vi "Teleop.vi"(10 "Match Info":T1={"Autonomous Elapsed Seconds"=0.0, "TeleOp Elapsed Seconds"=0.0, "Disabled Elapsed Seconds"=0.0, "Visited Autonomous"=FALSE, "Visited TeleOp"=FALSE, "Visited Disabled"=FALSE, "Autonomous Settings"={"Autonomous Style"=enum."Independent", "VI Refnum"=refnum}}, 11 "Call Context":T2) -> ()   [LabVIEW 2012]
doc: "This VI is called for each TeleOp packet received from the DS where the robot is not disabled. It is often used to read from the joysticks and update I/O or to update setpoints for timed control loops. It should complete and return within 20 milliseconds or it may miss DS packets."
uses:
  <vilib>/Rock Robotics/WPI/DriverStation/WPI_DriverStationDerivedRobotMode.ctl
  <vilib>/Rock Robotics/WPI/DriverStation/WPI_DriverStationMatch Info.ctl
  <vilib>/Rock Robotics/WPI/Relay/WPI_RelayValue.ctl
  Robot Global Data.vi
  <vilib>/Rock Robotics/WPI/Joystick/WPI_JoystickGetSetRefNum.vi
panel:
  in  "Ext Const":dbl=0.5
  in  "Dep Const":dbl=1.0
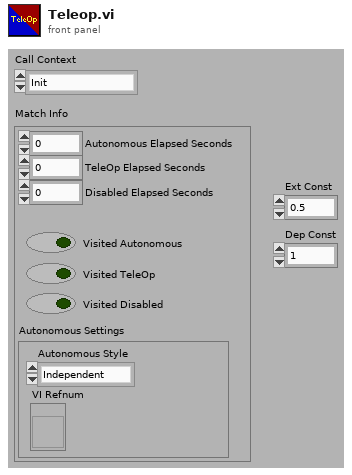
[diagram p1: front panel]
types:
  T1 = typedef "WPI_DriverStationMatch Info.ctl" = cluster{"Autonomous Elapsed Seconds":dbl, "TeleOp Elapsed Seconds":dbl, "Disabled Elapsed Seconds":dbl, "Visited Autonomous":bool, "Visited TeleOp":bool, "Visited Disabled":bool, "Autonomous Settings":cluster{"Autonomous Style":enum16{"Iterative", "Independent"}, "VI Refnum":refnum<vi>}}
  T2 = typedef "WPI_DriverStationDerivedRobotMode.ctl" = enum16{"Init", "Execute", "Stop"}
  T3 = typedef "WPI_RelayValue.ctl" = enum16{"Off", "On", "Forward", "Reverse"}
  T4 = cluster{"Driver Station Digital Input (1-8)[0]":bool, "Driver Station Digital Input (1-8)[1]":bool, "Driver Station Digital Input (1-8)[2]":bool, "Driver Station Digital Input (1-8)[3]":bool, "Driver Station Digital Input (1-8)[4]":bool, "Driver Station Digital Input (1-8)[5]":bool, "Driver Station Digital Input (1-8)[6]":bool, "Driver Station Digital Input (1-8)[7]":bool, "Driver Station Digital Input (1-8)[8]":bool}
  T5 = cluster{"Right Servo High":dbl, "Right Servo Mid":dbl, "Right Servo Low":dbl, "Left Servo High":dbl, "Left Servo Mid":dbl, "Left Servo Low":dbl}
  T6 = typedef "WPI_DigitalInputDevRef.ctl" = cluster{"DevStatus":errorcluster, "DIO Channel":T7, "Digital Module":T8}
  T7 = typedef "FPGA_DIOChannel.ctl" = enum8{"DIO 1", "DIO 2", "DIO 3", "DIO 4", "DIO 5", "DIO 6", "DIO 7", "DIO 8", "DIO 9", "DIO 10", "DIO 11", "DIO 12", "DIO 13", "DIO 14", "Invalid"}
  T8 = typedef "FPGA_TypedefDigitalModule.ctl" = enum16{"Digital Module 1", "Digital Module 2"}
  T9 = typedef "WPI_JoystickDevRef.ctl" = cluster{"Device":T10}
  T10 = typedef "WPI_JoystickDeviceEnum.ctl" = enum16{"USB 1", "USB 2", "USB 3", "USB 4", "Kinect 1", "Kinect 2"}
  T11 = cluster{"axis 1 (x)":dbl, "axis 2 (y)":dbl, "axis 3 (throttle)":dbl, "axis 4":dbl, "axis 5":dbl, "axis 6":dbl}
  T12 = typedef "WPI_RelayDevRef.ctl" = cluster{"DevStatus":errorcluster, "Relay Channel":T13, "Digital Module":T8, "Relay Direction":T14}
  T13 = typedef "FPGA_DIORelayChannel.ctl" = enum8{"Relay 1", "Relay 2", "Relay 3", "Relay 4", "Relay 5", "Relay 6", "Relay 7", "Relay 8", "Invalid"}
  T14 = typedef "WPI_RelayDirection.ctl" = enum16{"Both directions", "Forward only", "Reverse only"}
  T15 = typedef "WPI_ServoDeviceRef.ctl" = cluster{"DeviceStatus":errorcluster, "Digital Module":T8, "PWM Channel":T16, "DeadBand":T17}
  T16 = typedef "FPGA_DIOPWMChannel.ctl" = enum8{"PWM 1", "PWM 2", "PWM 3", "PWM 4", "PWM 5", "PWM 6", "PWM 7", "PWM 8", "PWM 9", "PWM 10", "Invalid"}
  T17 = typedef "WPI_PWMDeadband.ctl" = cluster{"Name":string, "maxPositivePwm":i32, "minPositivePwm":i32, "centerPwm":i32, "maxNegativePwm":i32, "minNegativePwm":i32, "angularRange":u16}
  T18 = typedef "WPI_MotorControlDeviceRef.ctl" = cluster{"DeviceStatus":errorcluster, "Type":enum16{"PWM", "CAN"}, "PWM":cluster{"Digital Module":T8, "PWM Channel":T16, "DeadBand":T17}, "CAN":cluster{"Device Number":u8, "Control Mode":T19, "Semaphore":T20, "Max Vout":dbl}, "Invert":bool, "TransformRef":T21, "InvTransformRef":T21}
  T19 = typedef "WPI_CANJaguar_ControlMode.ctl" = enum8{"Percent VBus", "Current", "Speed", "Position", "Voltage"}
  T20 = typedef "Semaphore RefNum" = refnum<k1>
  T21 = typedef "WPI_PWMTransform_ConPane.ctl" = refnum<vi>
  T22 = typedef "WPI_JoystickButtonState.ctl" = cluster{"Button 1":bool, "Button 2":bool, "Button 3":bool, "Button 4":bool, "Button 5":bool, "Button 6":bool, "Button 7":bool, "Button 8":bool, "Button 9":bool, "Button 10":bool, "Button 11":bool, "Button 12":bool}
  T23 = cluster{"FlipperLeftUp":dbl, "FlipperLeftDown":dbl, "FlipperRightUp":dbl, "FlipperRightDown":dbl, "KickerLeftBack":dbl, "KickerLeftForward":dbl, "KickerRightBack":dbl, "KickerRightForward":dbl}
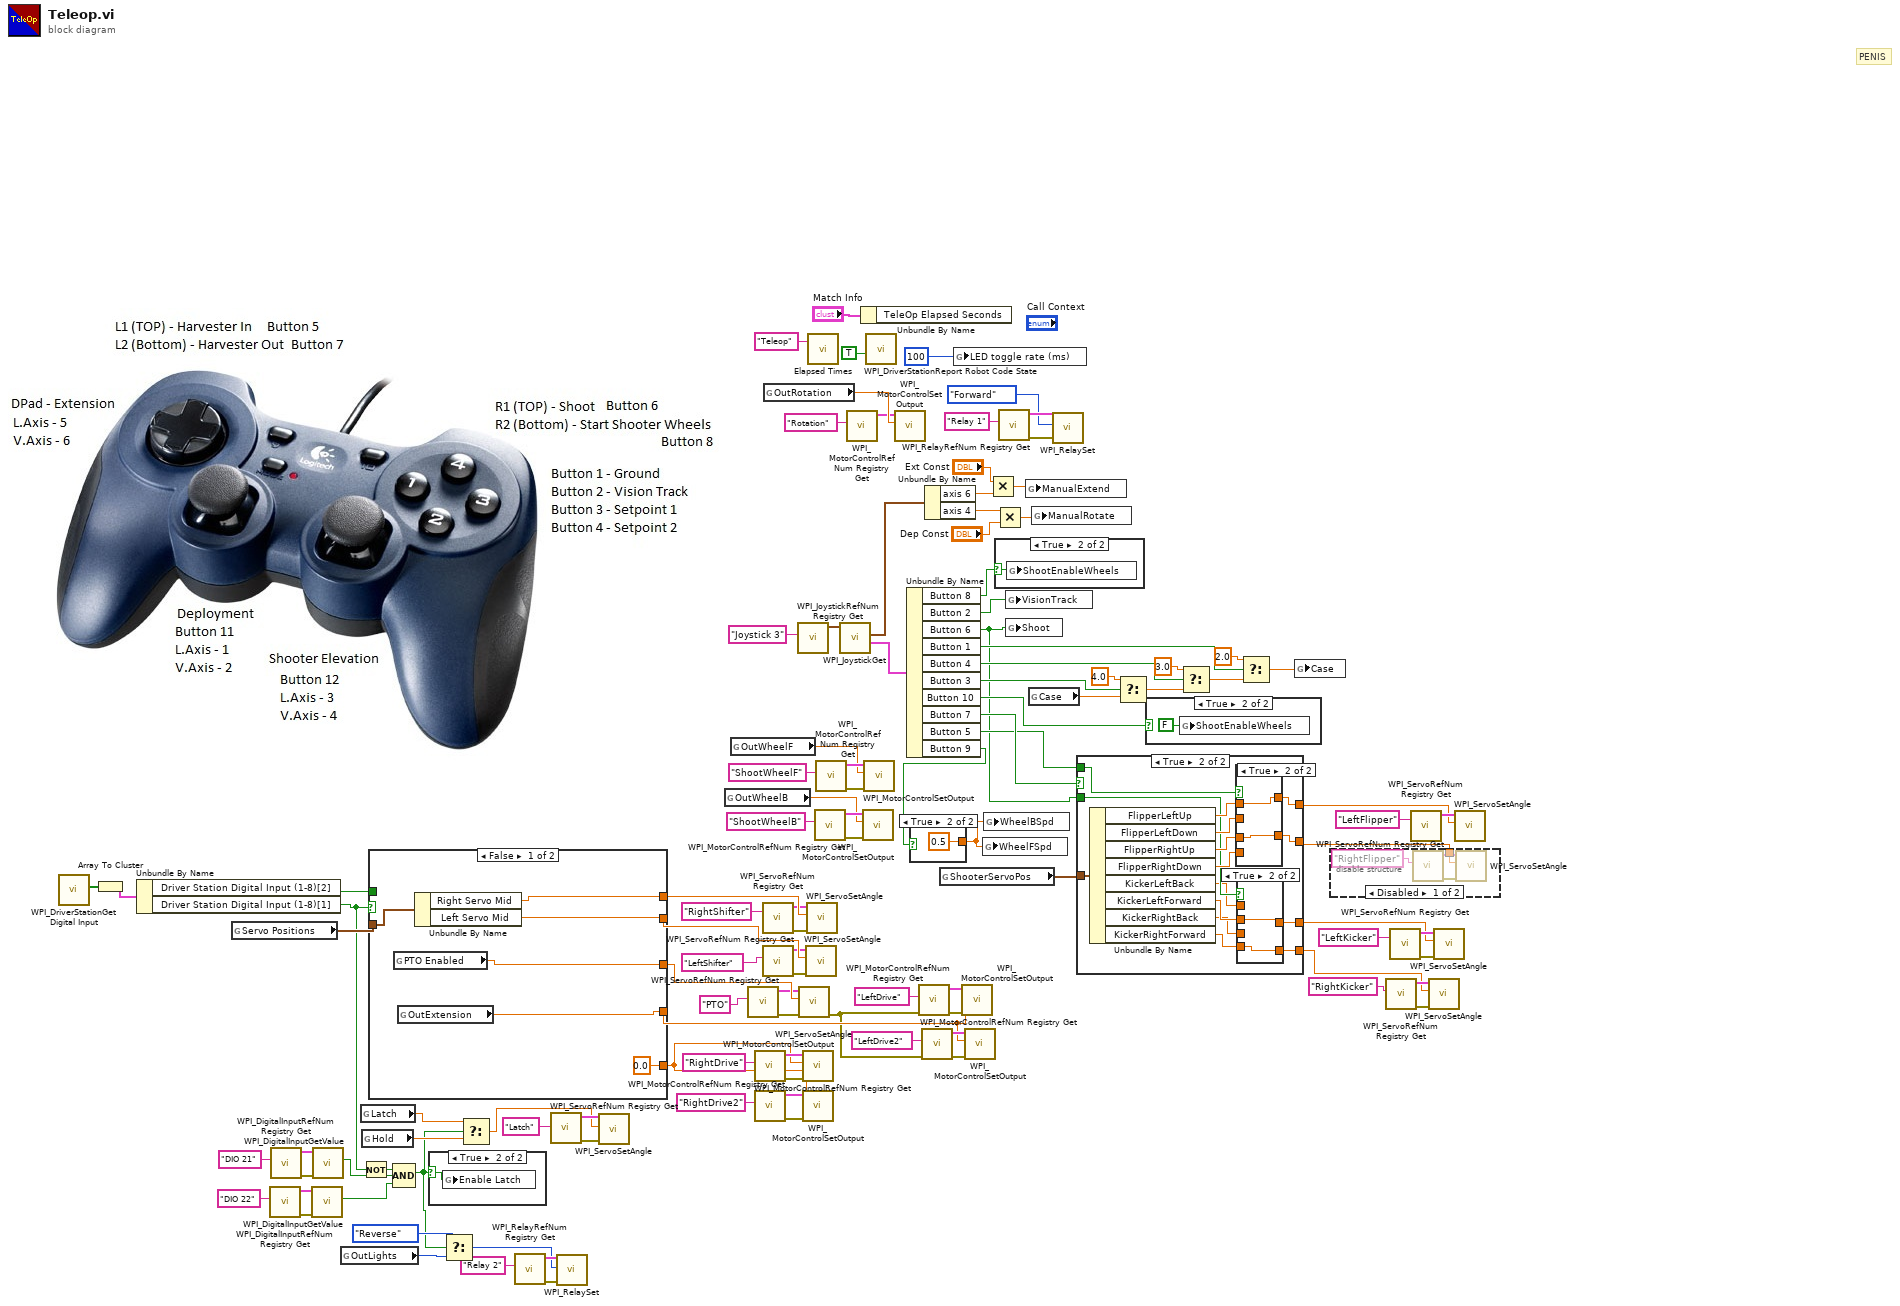
[diagram p0: block diagram]
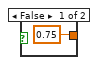
[diagram p2: hidden frame]
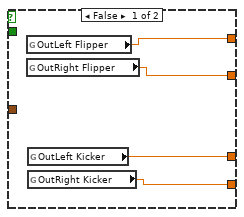
[diagram p4: hidden frame]
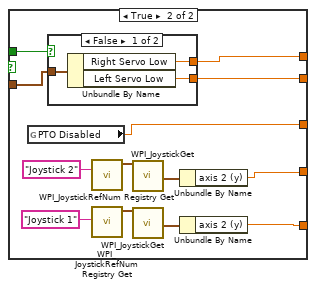
[diagram p8: hidden frame]
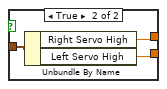
[diagram p9: hidden frame]
diagram:
  # "PENIS"
  n1 = call <vilib>:"WPI_DriverStationGet Digital Input.vi"() -> ("Driver Station Digital Input (1-8)"=w82:bool[])  [unwired: 11 in]
  n2 = Array To Cluster(array=w82) -> (cluster=w81:T4)
  n3 = Unbundle By Name(w81) -> ("Driver Station Digital Input (1-8)[2]"=w80:bool, "Driver Station Digital Input (1-8)[1]"=w41:bool)
  n4 = global read "Robot Global Data.vi" "Servo Positions"() -> (w79:T5)
  n5 = call <vilib>:"WPI_DigitalInputRefNum Registry Get.vi"("refnum name"="DIO 22") -> ("error out"=w5:errorcluster, "DigitalInputDevRef"=w6:T6)  [unwired: 9 in]
  n6 = call <vilib>:"WPI_DigitalInputRefNum Registry Get.vi"("refnum name"="DIO 21") -> ("error out"=w10:errorcluster, "DigitalInputDevRef"=w9:T6)  [unwired: 9 in]
  n7 = call <vilib>:"WPI_DigitalInputGetValue.vi"("error in (no error)"=w5, "DigitalInputDevRef"=w6) -> ("Value"=w2:bool)  [unwired: 7 in, 2 out]
  n8 = call <vilib>:"WPI_DigitalInputGetValue.vi"("error in (no error)"=w10, "DigitalInputDevRef"=w9) -> ("Value"=w3:bool)  [unwired: 7 in, 2 out]
  n9 = global read "Robot Global Data.vi" "OutLights"() -> (w47:T3)
  n10 = global read "Robot Global Data.vi" "Latch"() -> (w14:dbl)
  n11 = Not(x=w41) -> (.not. x?=w4:bool)
  n12 = global read "Robot Global Data.vi" "Hold"() -> (w13:dbl)
  n13 = case shown="False" w41 {
    tunnel: w80 -> [_ w133]
    tunnel: w79 -> [w120 w132]
    tunnel: [w119 w131] -> w78
    tunnel: [w118 w130] -> w77
    tunnel: [w117 w129] -> w70
    tunnel: [w115 w122] -> w69
    tunnel: [0.0 w121] -> w68
    frame False {
      n14 = global read "Robot Global Data.vi" "PTO Enabled"() -> (w117:dbl)
      n15 = global read "Robot Global Data.vi" "OutExtension"() -> (w115:dbl)
      n16 = Unbundle By Name(w120) -> ("Right Servo Mid"=w119:dbl, "Left Servo Mid"=w118:dbl)
    }
    frame True {
      n17 = global read "Robot Global Data.vi" "PTO Disabled"() -> (w129:dbl)
      n18 = case shown="False" w133 {
        tunnel: w132 -> [w136 w139]
        tunnel: [w135 w138] -> w131
        tunnel: [w134 w137] -> w130
        frame False {
          n19 = Unbundle By Name(w136) -> ("Right Servo Low"=w135:dbl, "Left Servo Low"=w134:dbl)
        }
        frame True {
          n20 = Unbundle By Name(w139) -> ("Right Servo High"=w138:dbl, "Left Servo High"=w137:dbl)
        }
      }
      n21 = call <vilib>:"WPI_JoystickRefNum Registry Get.vi"("refnum name"="Joystick 2") -> ("JoystickDevRef"=w123:T9)  [unwired: 1 in, 9 out]
      n22 = call <vilib>:"WPI_JoystickRefNum Registry Get.vi"("refnum name"="Joystick 1") -> ("JoystickDevRef"=w127:T9)  [unwired: 1 in, 9 out]
      n23 = call <vilib>:"WPI_JoystickGet.vi"("JoystickDevRef"=w123) -> ("Axes"=w125:T11)  [unwired: 1 in, 5 out]
      n24 = call <vilib>:"WPI_JoystickGet.vi"("JoystickDevRef"=w127) -> ("Axes"=w128:T11)  [unwired: 1 in, 5 out]
      n25 = Unbundle By Name(w125) -> ("axis 2 (y)"=w122:dbl)
      n26 = Unbundle By Name(w128) -> ("axis 2 (y)"=w121:dbl)
    }
  }
  n27 = Compound Arithmetic op=AND(w4, w3, w2) -> (w1:bool)
  n28 = case shown="True" w1 {
    selector: w1 -> [_ w140]
    frame False {
    }
    frame True {
      n29 = global write "Robot Global Data.vi" "Enable Latch"(w140) -> ()
    }
  }
  n30 = Select(t=WPI_RelayValue."Reverse" ("RelayValue"), s=w1, f=w47) -> (s? t:f=w45:T3)
  n31 = Select(t=w14, s=w1, f=w13) -> (s? t:f=w40:dbl)
  n32 = call <vilib>:"WPI_RelayRefNum Registry Get.vi"("refnum name"="Relay 2") -> ("error out"=w53:errorcluster, "RelayDevRef"=w51:T12)  [unwired: 9 in]
  n33 = call <vilib>:"WPI_ServoRefNum Registry Get.vi"("refnum name"="Latch") -> ("error out"=w44:errorcluster, "ServoDeviceRef"=w42:T15)  [unwired: 9 in]
  n34 = call <vilib>:"WPI_RelaySet.vi"("error in (no error)"=w53, "RelayValue"=w45, "RelayDevRef"=w51) -> ()  [unwired: 7 in, 2 out]
  n35 = call <vilib>:"WPI_ServoSetAngle.vi"("error in (no error)"=w44, "Angle"=w40, "ServoDeviceRef"=w42) -> ()  [unwired: 7 in, 2 out]
  n36 = global read "Robot Global Data.vi" "OutWheelB"() -> (w32:dbl)
  n37 = global read "Robot Global Data.vi" "OutWheelF"() -> (w33:dbl)
  n38 = call <vilib>:"WPI_ServoRefNum Registry Get.vi"("refnum name"="PTO") -> ("error out"=w63:errorcluster, "ServoDeviceRef"=w64:T15)  [unwired: 9 in]
  n39 = call <vilib>:"WPI_MotorControlRefNum Registry Get.vi"("refnum name"="RightDrive") -> ("error out"=w92:errorcluster, "MotorControlDevRef"=w94:T18)  [unwired: 9 in]
  n40 = call <vilib>:"WPI_MotorControlRefNum Registry Get.vi"("refnum name"="RightDrive2") -> ("error out"=w85:errorcluster, "MotorControlDevRef"=w83:T18)  [unwired: 9 in]
  n41 = call <vilib>:"WPI_ServoRefNum Registry Get.vi"("refnum name"="RightShifter") -> ("error out"=w73:errorcluster, "ServoDeviceRef"=w74:T15)  [unwired: 9 in]
  n42 = call <vilib>:"WPI_ServoRefNum Registry Get.vi"("refnum name"="LeftShifter") -> ("error out"=w75:errorcluster, "ServoDeviceRef"=w76:T15)  [unwired: 9 in]
  n43 = global read "Robot Global Data.vi" "OutRotation"() -> (w67:dbl)
  n44 = call <vilib>:"WPI_JoystickRefNum Registry Get.vi"("refnum name"="Joystick 3") -> ("JoystickDevRef"=w111:T9)  [unwired: 9 in, 1 out]
  n45 = call <vilib>:"WPI_ServoSetAngle.vi"("error in (no error)"=w63, "Angle"=w70, "ServoDeviceRef"=w64) -> ("error out"=w59:errorcluster)  [unwired: 7 in, 1 out]
  n46 = call <vilib>:"WPI_MotorControlSetOutput.vi"("error in (no error)"=w92, "Output"=w68, "MotorControlDevRef"=w94) -> ()  [unwired: 6 in, 3 out]
  n47 = call <vilib>:"WPI_MotorControlSetOutput.vi"("error in (no error)"=w85, "Output"=w68, "MotorControlDevRef"=w83) -> ()  [unwired: 6 in, 3 out]
  n48 = call <vilib>:"WPI_ServoSetAngle.vi"("error in (no error)"=w75, "Angle"=w77, "ServoDeviceRef"=w76) -> ()  [unwired: 7 in, 2 out]
  n49 = call <vilib>:"WPI_ServoSetAngle.vi"("error in (no error)"=w73, "Angle"=w78, "ServoDeviceRef"=w74) -> ()  [unwired: 7 in, 2 out]
  n50 = call "Elapsed Times.vi"("Call Name"="Teleop") -> ()  [unwired: 2 in, 1 out]
  n51 = call <vilib>:"WPI_MotorControlRefNum Registry Get.vi"("refnum name"="ShootWheelB") -> ("error out"=w35:errorcluster, "MotorControlDevRef"=w36:T18)  [unwired: 9 in]
  n52 = call <vilib>:"WPI_MotorControlRefNum Registry Get.vi"("refnum name"="ShootWheelF") -> ("error out"=w37:errorcluster, "MotorControlDevRef"=w34:T18)  [unwired: 9 in]
  n53 = call <vilib>:"WPI_JoystickGet.vi"("JoystickDevRef"=w111) -> ("Buttons"=w109:T22, "Axes"=w108:T11)  [unwired: 4 in, 1 out]
  n54 = call <vilib>:"WPI_MotorControlRefNum Registry Get.vi"("refnum name"="Rotation") -> ("MotorControlDevRef"=w65:T18)  [unwired: 9 in, 1 out]
  n55 = Unbundle By Name("Match Info") -> ()  [unwired: 1 out]
  n56 = call <vilib>:"WPI_MotorControlSetOutput.vi"("error in (no error)"=w35, "Output"=w32, "MotorControlDevRef"=w36) -> ()  [unwired: 6 in, 3 out]
  n57 = call <vilib>:"WPI_MotorControlSetOutput.vi"("error in (no error)"=w37, "Output"=w33, "MotorControlDevRef"=w34) -> ()  [unwired: 6 in, 3 out]
  n58 = call <vilib>:"WPI_DriverStationReport Robot Code State.vi"("TeleOp"=TRUE ("Autonomous")) -> ()  [unwired: 10 in, 1 out]
  n59 = call <vilib>:"WPI_MotorControlSetOutput.vi"("Output"=w67, "MotorControlDevRef"=w65) -> ()  [unwired: 7 in, 3 out]
  n60 = Unbundle By Name(w109) -> ("Button 8"=w96:bool, "Button 2"=w107:bool, "Button 6"=w16:bool, "Button 1"=w106:bool, "Button 4"=w104:bool, "Button 3"=w103:bool, "Button 10"=w31:bool, "Button 7"=w30:bool, "Button 5"=w29:bool, "Button 9"=w11:bool)
  n61 = case shown="True" w11 {
    tunnel: [0.75 0.5] -> w12
    frame False {
    }
    frame True {
    }
  }
  n62 = call <vilib>:"WPI_MotorControlRefNum Registry Get.vi"("error in (no error)"=w59, "refnum name"="LeftDrive") -> ("error out"=w87:errorcluster, "MotorControlDevRef"=w90:T18)  [unwired: 8 in]
  n63 = call <vilib>:"WPI_MotorControlRefNum Registry Get.vi"("error in (no error)"=w59, "refnum name"="LeftDrive2") -> ("error out"=w86:errorcluster, "MotorControlDevRef"=w88:T18)  [unwired: 8 in]
  n64 = Unbundle By Name(w108) -> ("axis 6"=w50:dbl, "axis 4"=w60:dbl)
  n65 = global read "Robot Global Data.vi" "ShooterServoPos"() -> (w17:T23)
  n66 = global write "Robot Global Data.vi" "LED toggle rate (ms)"(u32 100 ("LED ms toggle rate")) -> ()
  n67 = call <vilib>:"WPI_MotorControlSetOutput.vi"("error in (no error)"=w87, "Output"=w69, "MotorControlDevRef"=w90) -> ()  [unwired: 6 in, 3 out]
  n68 = call <vilib>:"WPI_MotorControlSetOutput.vi"("error in (no error)"=w86, "Output"=w69, "MotorControlDevRef"=w88) -> ()  [unwired: 6 in, 3 out]
  n69 = global write "Robot Global Data.vi" "WheelFSpd"(w12) -> ()
  n70 = global write "Robot Global Data.vi" "WheelBSpd"(w12) -> ()
  n71 = Multiply(x="Ext Const", y=w50) -> (x*y=w48:dbl)
  n72 = Multiply(x=w60, y="Dep Const") -> (x*y=w58:dbl)
  n73 = case shown="True" w96 {
    selector: w96 -> [_ w143]
    frame False {
    }
    frame True {
      n74 = global write "Robot Global Data.vi" "ShootEnableWheels"(w143) -> ()
    }
  }
  n75 = call <vilib>:"WPI_RelayRefNum Registry Get.vi"("refnum name"="Relay 1") -> ("error out"=w55:errorcluster, "RelayDevRef"=w57:T12)  [unwired: 9 in]
  n76 = global write "Robot Global Data.vi" "VisionTrack"(w107) -> ()
  n77 = global write "Robot Global Data.vi" "Shoot"(w16) -> ()
  n78 = global write "Robot Global Data.vi" "ManualExtend"(w48) -> ()
  n79 = global read "Robot Global Data.vi" "Case"() -> (w98:dbl)
  n80 = global write "Robot Global Data.vi" "ManualRotate"(w58) -> ()
  n81 = call <vilib>:"WPI_RelaySet.vi"("error in (no error)"=w55, "RelayValue"=WPI_RelayValue."Forward", "RelayDevRef"=w57) -> ()  [unwired: 7 in, 2 out]
  n82 = case shown="True" w30 {
    tunnel: w29 -> [_ w148]
    tunnel: [w147 w161] -> w20
    tunnel: [w146 w159] -> w19
    tunnel: [w145 w150] -> w18
    tunnel: [w144 w149] -> w15
    tunnel: w17 -> [_ w162]
    tunnel: w16 -> [_ w155]
    frame False {
      n83 = global read "Robot Global Data.vi" "OutLeft Flipper"() -> (w147:dbl)
      n84 = global read "Robot Global Data.vi" "OutRight Flipper"() -> (w146:dbl)
      n85 = global read "Robot Global Data.vi" "OutLeft Kicker"() -> (w145:dbl)
      n86 = global read "Robot Global Data.vi" "OutRight Kicker"() -> (w144:dbl)
    }
    frame True {
      n87 = Unbundle By Name(w162) -> ("FlipperLeftUp"=w160:dbl, "FlipperLeftDown"=w157:dbl, "FlipperRightUp"=w158:dbl, "FlipperRightDown"=w156:dbl, "KickerLeftBack"=w154:dbl, "KickerLeftForward"=w153:dbl, "KickerRightBack"=w152:dbl, "KickerRightForward"=w151:dbl)
      n88 = case shown="True" w148 {
        tunnel: [w168 w170] -> w161
        tunnel: w160 -> [_ w170]
        tunnel: [w167 w169] -> w159
        tunnel: w158 -> [_ w169]
        tunnel: w157 -> [w168 _]
        tunnel: w156 -> [w167 _]
        frame False {
        }
        frame True {
        }
      }
      n89 = case shown="True" w155 {
        tunnel: w154 -> [w164 _]
        tunnel: w153 -> [_ w165]
        tunnel: w152 -> [w163 _]
        tunnel: w151 -> [_ w166]
        tunnel: [w164 w165] -> w150
        tunnel: [w163 w166] -> w149
        frame False {
        }
        frame True {
        }
      }
    }
  }
  n90 = Select(t=4.0, s=w103, f=w98) -> (s? t:f=w102:dbl)
  n91 = case shown="True" w31 {
    frame False {
    }
    frame True {
      n92 = global write "Robot Global Data.vi" "ShootEnableWheels"(FALSE ("ShootStartWheels")) -> ()
    }
  }
  n93 = Select(t=3.0, s=w104, f=w102) -> (s? t:f=w100:dbl)
  n94 = Select(t=2.0, s=w106, f=w100) -> (s? t:f=w97:dbl)
  n95 = global write "Robot Global Data.vi" "Case"(w97) -> ()
  n96 = disable-structure shown="Disabled" {
    disable-tunnel: w19 -> [w172 _]
    frame Disabled {
      n97 = call <vilib>:"WPI_ServoRefNum Registry Get.vi"("refnum name"="RightFlipper") -> ("error out"=w175:errorcluster, "ServoDeviceRef"=w173:T15)  [unwired: 9 in]
      n98 = call <vilib>:"WPI_ServoSetAngle.vi"("error in (no error)"=w175, "Angle"=w172, "ServoDeviceRef"=w173) -> ()  [unwired: 7 in, 2 out]
    }
    frame Enabled {
    }
  }
  n99 = call <vilib>:"WPI_ServoRefNum Registry Get.vi"("refnum name"="RightKicker") -> ("error out"=w27:errorcluster, "ServoDeviceRef"=w25:T15)  [unwired: 9 in]
  n100 = call <vilib>:"WPI_ServoRefNum Registry Get.vi"("refnum name"="LeftKicker") -> ("error out"=w21:errorcluster, "ServoDeviceRef"=w22:T15)  [unwired: 9 in]
  n101 = call <vilib>:"WPI_ServoRefNum Registry Get.vi"("refnum name"="LeftFlipper") -> ("ServoDeviceRef"=w23:T15)  [unwired: 9 in, 1 out]
  n102 = call <vilib>:"WPI_ServoSetAngle.vi"("error in (no error)"=w27, "Angle"=w15, "ServoDeviceRef"=w25) -> ()  [unwired: 7 in, 2 out]
  n103 = call <vilib>:"WPI_ServoSetAngle.vi"("error in (no error)"=w21, "Angle"=w18, "ServoDeviceRef"=w22) -> ()  [unwired: 7 in, 2 out]
  n104 = call <vilib>:"WPI_ServoSetAngle.vi"("Angle"=w20, "ServoDeviceRef"=w23) -> ()  [unwired: 8 in, 2 out]
